vi "xy chart buffer (subVI).vi"(6 "remove nan? (T)":bool=TRUE, 8 "initialize buffer? (F)":bool, 9 "buffer length (50)":i32=50, 10 "new xy point []":cluster{"x":dbl, "y":dbl}[](array[cluster])) -> (3 "xy chart data []":cluster{"x":dbl[], "y":dbl[]}[](array[cluster]))   [LabVIEW 2021]
panel:
  out "xy chart data [] buffer":cluster{"x":dbl[], "y":dbl[]}[](array[cluster])
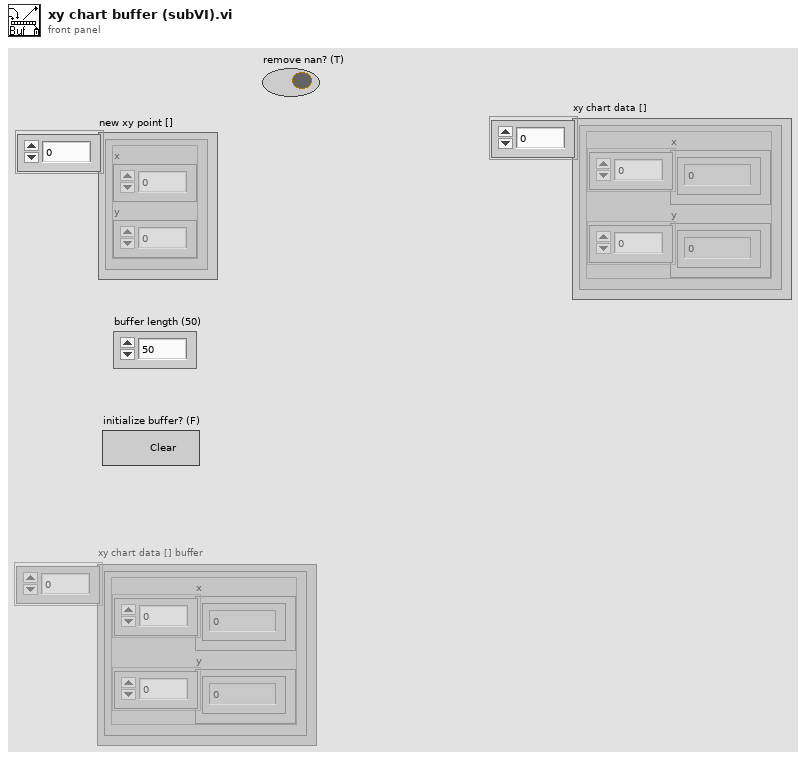
[diagram p1: front panel]
types:
  T1 = cluster{"filtered array":dbl[], "filtered array":dbl[]}
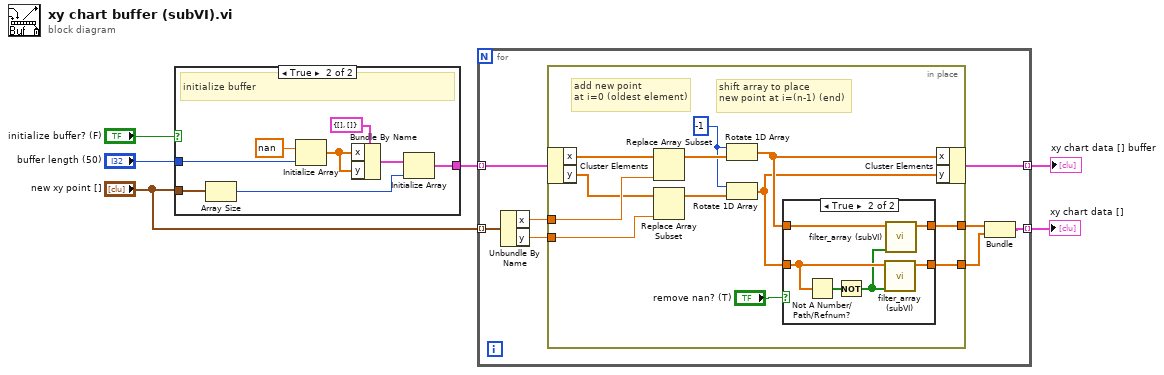
[diagram p0: block diagram]
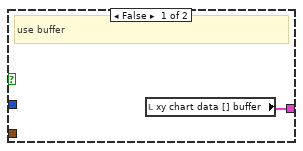
[diagram p3: hidden frame]
diagram:
  n1 = case shown="True" "initialize buffer? (F)" {
    tunnel: [w7 w12] -> w5
    tunnel: "buffer length (50)" -> [_ w11]
    tunnel: "new xy point []" -> [_ w9]
    frame False {
      # "use buffer"
      n2 = local read "xy chart data [] buffer"() -> (w7:cluster{"x":dbl[], "y":dbl[]}[])
    }
    frame True {
      # "initialize buffer"
      n3 = Array Size(array=w9) -> (size(s)=w8:i32)
      n4 = Initialize Array(nan ("element"), w11) -> (w14:dbl[])
      n5 = Bundle By Name(cluster=cluster{"x":dbl[], "y":dbl[]} {"x"=[], "y"=[]} ("XY Chart Data"), "x"=w14, "y"=w14) -> (w13:cluster{"x":dbl[], "y":dbl[]})
      n6 = Initialize Array(w13, w8) -> (w12:cluster{"x":dbl[], "y":dbl[]}[])
    }
  }
  n7 = for {
    tunnel: "new xy point []" -> [w23] mode=indexing
    tunnel: w5 -> [w20] mode=indexing
    tunnel: [w19] -> w2 mode=indexing
    tunnel: [w16] -> w1 mode=indexing
    n8 = Unbundle By Name(w23) -> ("x"=w22:dbl, "y"=w21:dbl)
    n9 = in-place "In Place Element Structure" {
      in-place-border: w22 -> [w35]
      in-place-border: w21 -> [w34]
      in-place-border: [w28] -> w17
      in-place-border: [w27] -> w18
      w31 = -1 ("n")
      # "shift array to place \nnew point at i=(n-1) (end)"
      # "add new point \nat i=0 (oldest element)"
      n10 = in-place-cluster #1(w20) -> ("x"=w30:dbl[], "y"=w29:dbl[])
      n11 = Replace Array Subset(array=w30, new element=w35) -> (w32:dbl[])  [unwired: 1 in]
      n12 = Replace Array Subset(array=w29, new element=w34) -> (w33:dbl[])  [unwired: 1 in]
      n13 = Rotate 1D Array(1:w32, 2:w31) -> (0:w26:dbl[])
      n14 = Rotate 1D Array(1:w33, 2:w31) -> (0:w25:dbl[])
      n15 = case shown="True" "remove nan? (T)" {
        tunnel: [w36 w43] -> w28
        tunnel: [w37 w42] -> w27
        tunnel: w26 -> [w36 w41]
        tunnel: w25 -> [w37 w40]
        frame False {
        }
        frame True {
          n16 = Not A Number/Path/Refnum?(number/path/refnum=w40) -> (NaN/Path/Refnum?=w39:bool[])
          n17 = Not(x=w39) -> (.not. x?=w38:bool[])
          n18 = call "filter_array (subVI).vi"("filter"=w38, "array"=w40) -> ("filtered array"=w42:dbl[])  [unwired: 9 in]
          n19 = call "filter_array (subVI).vi"("filter"=w38, "array"=w41) -> ("filtered array"=w43:dbl[])  [unwired: 9 in]
        }
      }
      n20 = in-place-cluster #1("x"=w26, "y"=w25) -> (w19:cluster{"x":dbl[], "y":dbl[]})
    }
    n21 = Bundle("filtered array"=w17, "filtered array"=w18) -> (w16:T1)  [unwired: 1 in]
  }
  "xy chart data [] buffer" <- w2
  "xy chart data []" <- w1
